vi "Create Waveform Cluster (2D).vi"(1 "dx":dbl, 2 "Array":dbl[][](array[numeric]), 4 "Offset":dbl) -> (5 "waveform cluster":cluster{"offset":dbl, "dx":dbl, "Y":dbl[][]})   [LabVIEW 2020]
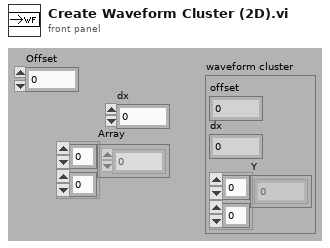
[diagram p1: front panel]
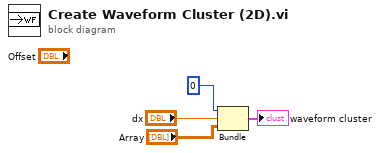
[diagram p0: block diagram]
diagram:
  n1 = Bundle(0, "dx"="dx", "Array"="Array") -> (→"waveform cluster":cluster{i32, "dx":dbl, "Array":dbl[][]})  [unwired: 1 in]
